vi "price.vi"(8 "error in (no error)":errorcluster, 11 "ChickenBurger in":refnum<class "ChickenBurger.lvclass">) -> (0 "error out":errorcluster, 2 "price":dbl, 3 "ChickenBurger out":refnum<class "ChickenBurger.lvclass">)   [LabVIEW 2018, in "ChickenBurger.lvclass"]
uses:
  ChickenBurger.lvclass
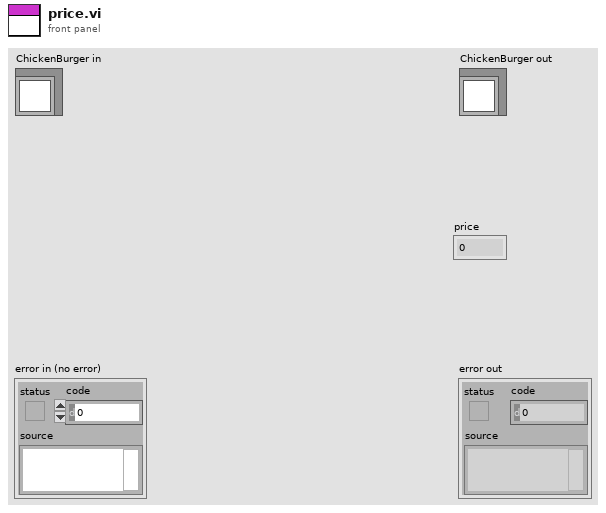
[diagram p1: front panel]
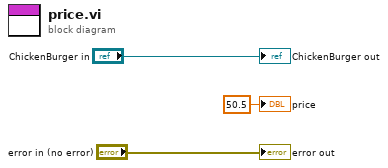
[diagram p0: block diagram]
diagram:
  "error out" <- "error in (no error)"
  "ChickenBurger out" <- "ChickenBurger in"
  "price" <- 50.5 ("price")
